vi "IncrementPosition.vi"(0 "VISA resource name":refnum<visa-resource-name>, 1 "error in (no error)":errorcluster) -> (2 "VISA resource name out":refnum<visa-resource-name>, 3 "Command not accepted":bool, 4 "error out":errorcluster)   [LabVIEW 2017, in "Spectral Products CM110.lvlib"]
uses:
  Spectral Products CM110.lvlib
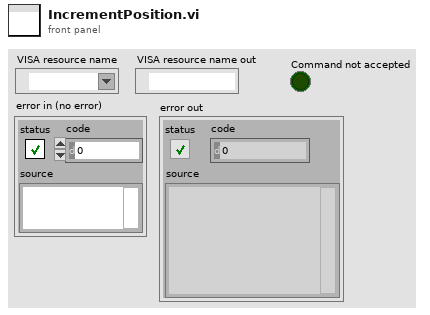
[diagram p1: front panel]
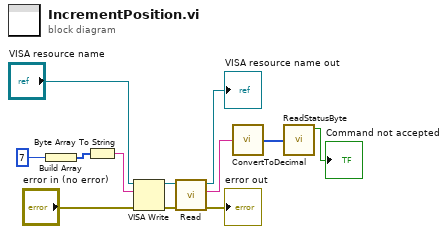
[diagram p0: block diagram]
diagram:
  n1 = Build Array(u8 7 ("element")) -> (w5:u8[])
  n2 = Byte Array To String(unsigned byte array=w5) -> (string=w4:string)
  n3 = VISA Write(VISA resource name="VISA resource name", write buffer=w4, error in (no error)="error in (no error)") -> (VISA resource name out=w11:refnum<visa-resource-name>, error out=w12:errorcluster)  [unwired: 1 out]
  n4 = call "Read.vi"("error in (no error)"=w12, "VISA Refnum in"=w11) -> ("error out"=→"error out":errorcluster, "read buffer"=w6:string, "VISA Refnum out"=→"VISA resource name out":refnum<visa-resource-name>)  [unwired: 6 in, 1 out]
  n5 = call "ConvertToDecimal.vi"("read buffer"=w6) -> ("unsigned byte array"=w2:u8[])
  n6 = call "ReadStatusByte.vi"("unsigned byte array"=w2) -> ("Command not accepted"=→"Command not accepted":bool)  [unwired: 4 in, 5 out]
